vi "p8.5.vi"() -> ()   [LabVIEW 2020]
uses:
  <vilib>/vision/NI_Vision_Development_Module.lvlib
panel:
  out "FFT imagen1":T1(plugin-control)
  in  "FFT Image Type 2":T2=3 items=["Grayscale (U8)", "Grayscale (I16)", "Grayscale (SGL)", "Complex (CSG)", "RGB (U32)", "HSL (U32)", "RGB (U64)", "Grayscale (U16)"]
  in  "Image Type":T2 items=["Grayscale (U8)", "Grayscale (I16)", "Grayscale (SGL)", "Complex (CSG)", "RGB (U32)", "HSL (U32)", "RGB (U64)", "Grayscale (U16)"]
  out "Imagen1":T1(plugin-control)
  in  "File Path":path=path "Z:/BenoBelmont/teleco2020_21/TDS/laboratorio/P789/imagenes_monocromas/lenna_mono.tif"
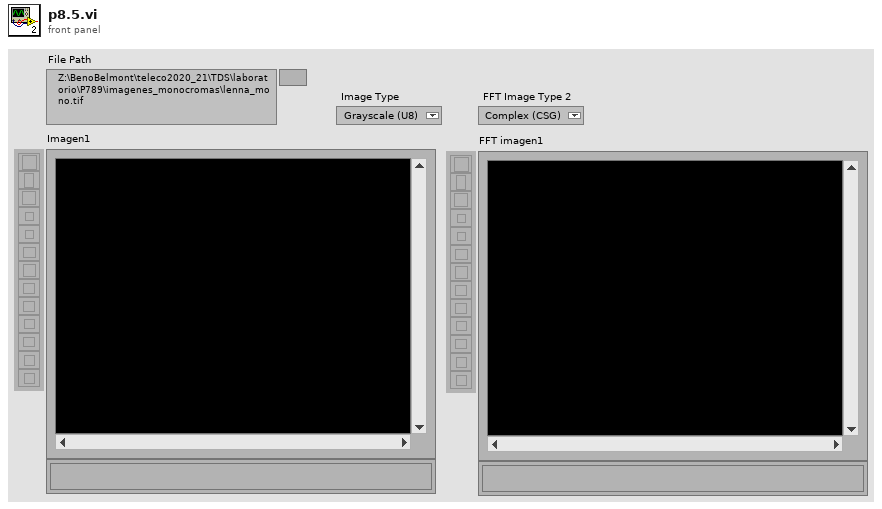
[diagram p1: front panel]
types:
  T1 = typedef "IMAQ Image.ctl" = refnum<image>
  T2 = typedef "Image Type" = u32
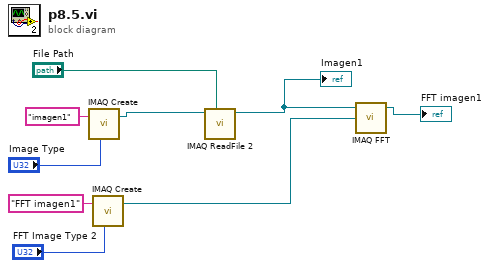
[diagram p0: block diagram]
diagram:
  n1 = call "IMAQ Create"("Image Name"="imagen1", "Image Type"="Image Type") -> ("New Image"=w9:T1)  [unwired: 3 in, 1 out]
  n2 = call "IMAQ Create"("Image Name"="FFT imagen1", "Image Type"="FFT Image Type 2") -> ("New Image"=w2:T1)  [unwired: 3 in, 1 out]
  n3 = call "IMAQ ReadFile 2"("File Path"="File Path", "Image"=w9) -> ("Image Out"=w5:T1)  [unwired: 5 in, 4 out]
  "Imagen1" <- w5
  n4 = call "IMAQ FFT"("Image Dst"=w2, "Image Src"=w5) -> ("Image Dst Out"=→"FFT imagen1":T1)  [unwired: 2 in, 1 out]
